vi "Get Network Interfaces Info.vi"(8 "Error In":errorcluster, 11 "Install LV Data":T3={"SSH Session"=refnum, "Status Log"="", "Detailed Log"="", "Credentials"={"Hostname or IP"="192.168.7.2", "Username"="root", "Password"=""}, "Target Info"={"OS Version"="", "CPU"="", "Systemd Version"="", "Internet Access"=FALSE, "Device Type"="", "LV Installed Ver"="", "LV Available Ver"="", "LV Upgrade Available"=FALSE, "Hostname"="", "NIC Info"=[]}, "Reboot Required?"=FALSE}) -> (0 "Error Out":errorcluster, 3 "Install LV Data":T3={"SSH Session"=refnum, "Status Log"="", "Detailed Log"="", "Credentials"={"Hostname or IP"="192.168.7.2", "Username"="root", "Password"=""}, "Target Info"={"OS Version"="", "CPU"="", "Systemd Version"="", "Internet Access"=FALSE, "Device Type"="", "LV Installed Ver"="", "LV Available Ver"="", "LV Upgrade Available"=FALSE, "Hostname"="", "NIC Info"=[]}, "Reboot Required?"=FALSE})   [LabVIEW 2014, in "LMH-LINX.lvlib"]
uses:
  <vilib>/MakerHub/LINX/LMH-LINX.lvlib
  <vilib>/MakerHub/LINX/Private/Utilties/Target Management/Install LV Data.ctl
  C:/Program Files (x86)/National Instruments/LabVIEW 2014/vi.lib/MakerHub/LINX/Resources/Renci.SshNet.dll
  Resources/Renci.SshNet.dll
  <vilib>/MakerHub/LINX/Private/Utilties/Target Management/Target Info.ctl
  <vilib>/MakerHub/LINX/Private/Utilties/Target Management/NIC Info.ctl
  <vilib>/MakerHub/LINX/Private/Utilties/Target Management/NIC Mode.ctl
panel:
  out "Target Info.NIC Info":T1[](array[typedef])
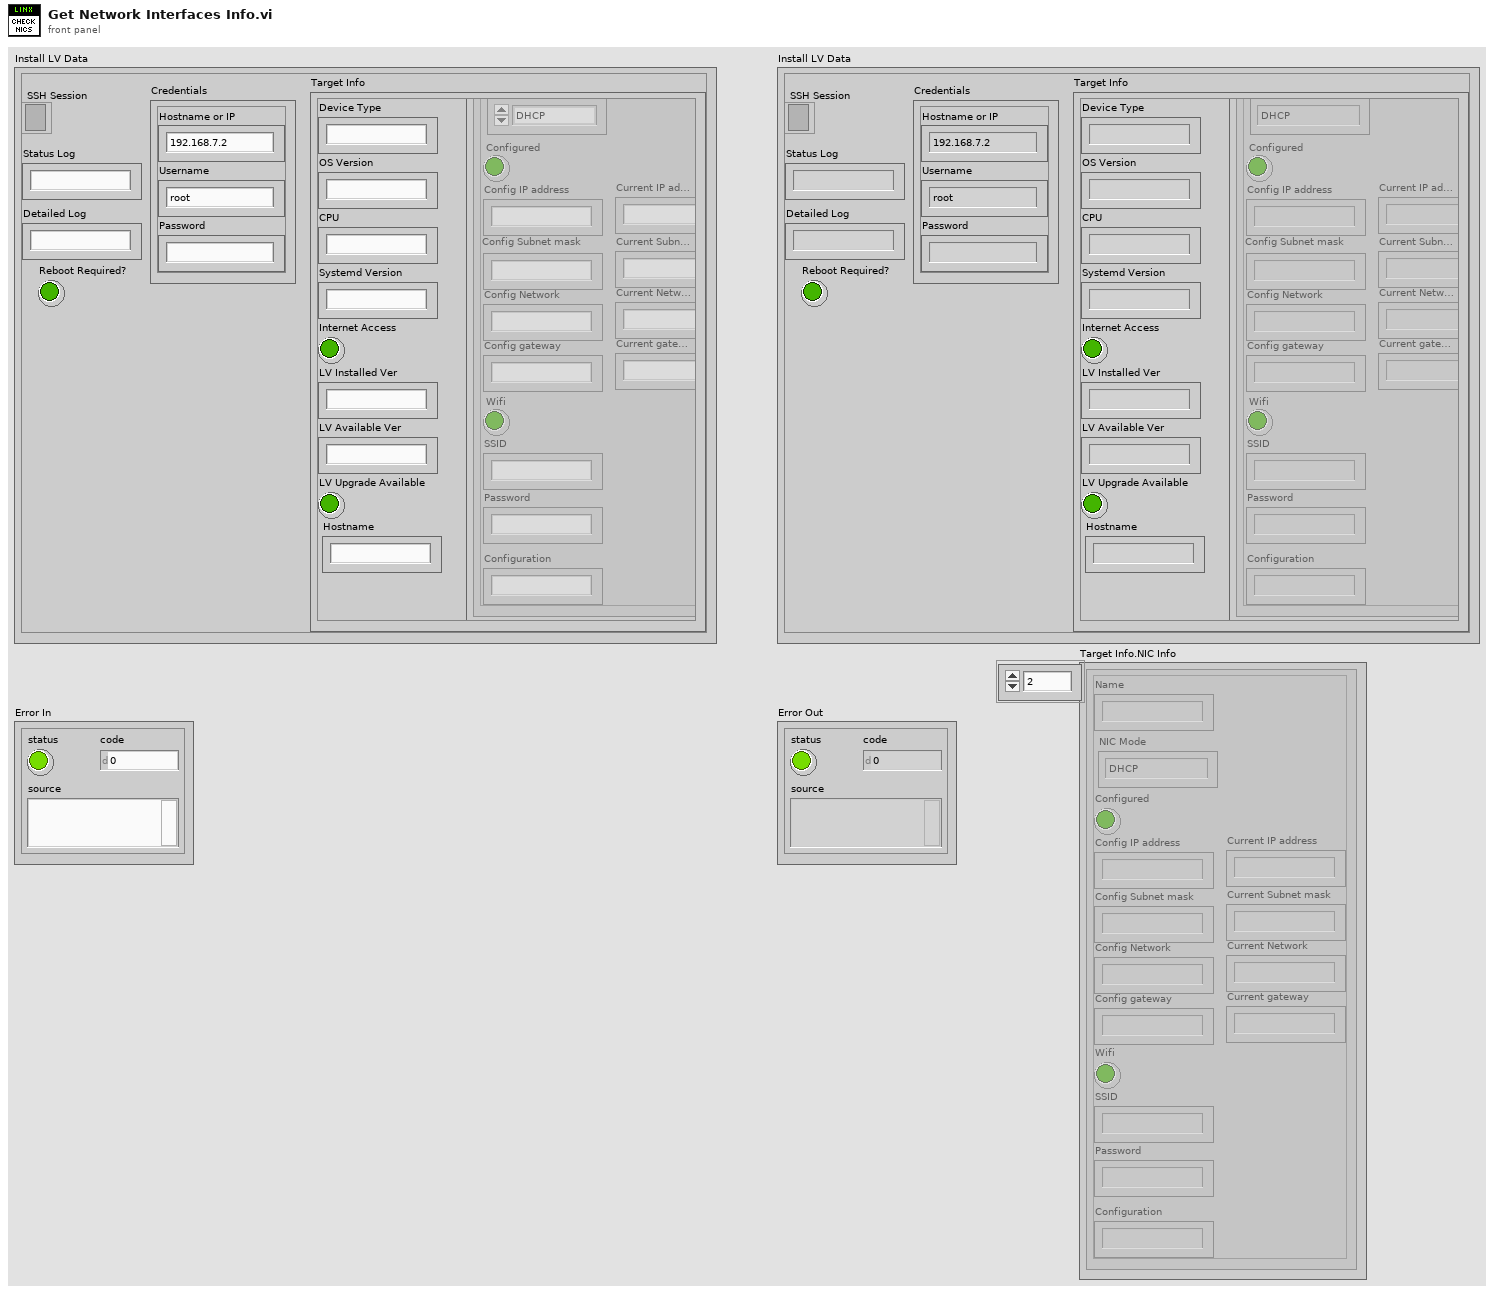
[diagram p1: front panel]
types:
  T1 = typedef "LMH-LINX.lvlib/NIC Info.ctl" = cluster{"Name":string, "NIC Mode":T2, "Configured":bool, "Config IP address":string, "Config Subnet mask":string, "Config Network":string, "Config gateway":string, "Wifi":bool, "SSID":string, "Password":string, "Configuration":string, "Current IP address":string, "Current Subnet mask":string, "Current gateway":string, "Current Network":string}
  T2 = typedef "LMH-LINX.lvlib/NIC Mode.ctl" = enum16{"DHCP", "Static", "Loopback"}
  T3 = typedef "LMH-LINX.lvlib/Install LV Data.ctl" = cluster{"SSH Session":refnum<k24>, "Status Log":string, "Detailed Log":string, "Credentials":cluster{"Hostname or IP":string, "Username":string, "Password":string}, "Target Info":T4, "Reboot Required?":bool}
  T4 = typedef "LMH-LINX.lvlib/Target Info.ctl" = cluster{"OS Version":string, "CPU":string, "Systemd Version":string, "Internet Access":bool, "Device Type":string, "LV Installed Ver":string, "LV Available Ver":string, "LV Upgrade Available":bool, "Hostname":string, "NIC Info":T1[]}
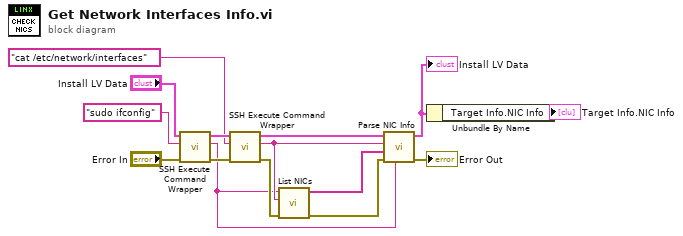
[diagram p0: block diagram]
diagram:
  n1 = call <vilib>:"SSH Execute Command Wrapper.vi"("Error In"="Error In", "Command"="sudo ifconfig", "Install LV Data in"="Install LV Data") -> ("Error Out"=w3:errorcluster, "Std Out"=w1:string, "Install LV Data out"=w11:T3)  [unwired: 6 in]
  n2 = call <vilib>:"SSH Execute Command Wrapper.vi"("Error In"=w3, "Command"="cat /etc/network/interfaces", "Install LV Data in"=w11) -> ("Error Out"=w4:errorcluster, "Std Out"=w6:string, "Install LV Data out"=w9:T3)  [unwired: 6 in]
  n3 = call <vilib>:"List NICs.vi"("Error In"=w4, "Network Interface Config"=w6, "ifconfig"=w1) -> ("Error Out"=w2:errorcluster, "All NICs"=w14:string[])  [unwired: 7 in]
  n4 = call <vilib>:"Parse NIC Info.vi"("ifconfig"=w1, "Error In"=w2, "All NICs"=w14, "interfaces config"=w6, "Install LV Data"=w9) -> ("Error Out"=→"Error Out":errorcluster, "Install LV Data"=w5:T3)  [unwired: 5 in]
  "Install LV Data" <- w5
  n5 = Unbundle By Name(w5) -> ("Target Info.NIC Info"=→"Target Info.NIC Info":T1[])
